vi "StateMachine.vi"() -> ()   [LabVIEW 2017]
uses:
  StateMachineControl.ctl
  global_output.vi
  IR_global.vi
  global_stop.vi
panel:
  in  "Go":bool
  out "State":T1
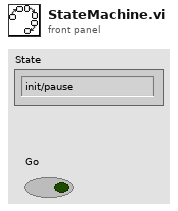
[diagram p1: front panel]
types:
  T1 = typedef "StateMachineControl.ctl" = enum16{"init/pause", "waypoint A", "wait at A", "waypoint B", "wait at B"}
  T2 = typedef "StateMachineControl.ctl" = enum16{"init/pause", "forward", "left", "right", "continue left", "continue right", "shutdown"}
  T3 = enum16{"Forward", "Backward", "Left", "Right", "Rotate Left", "Rotate Right"}
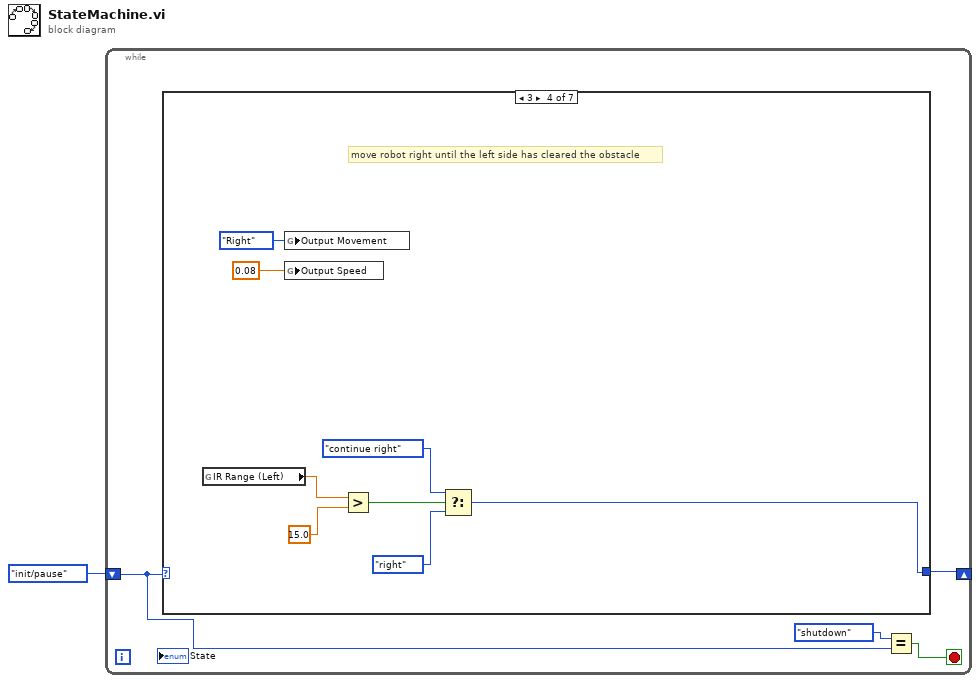
[diagram p0: block diagram]
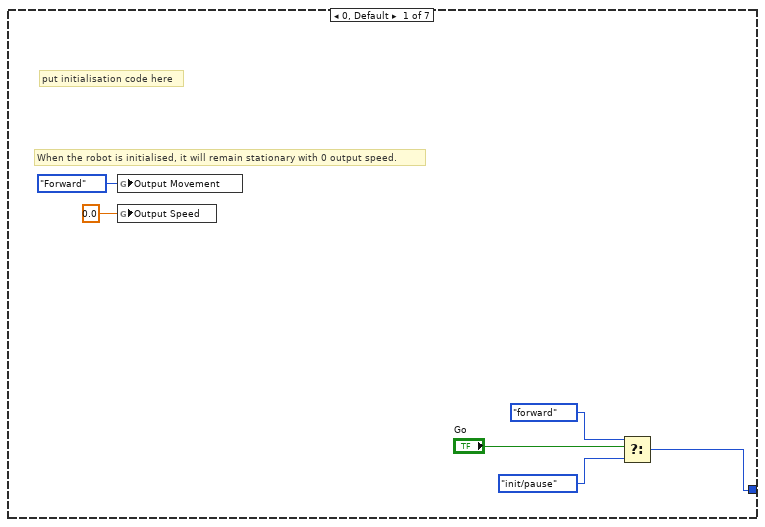
[diagram p2: hidden frame]
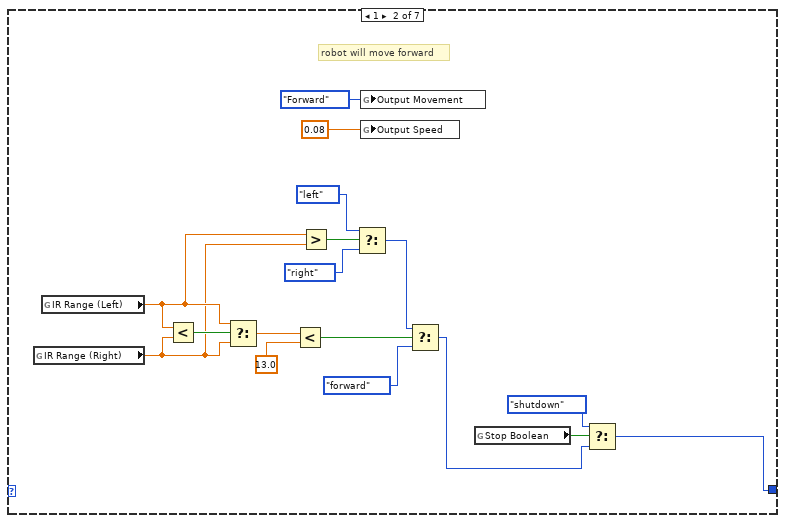
[diagram p3: hidden frame]
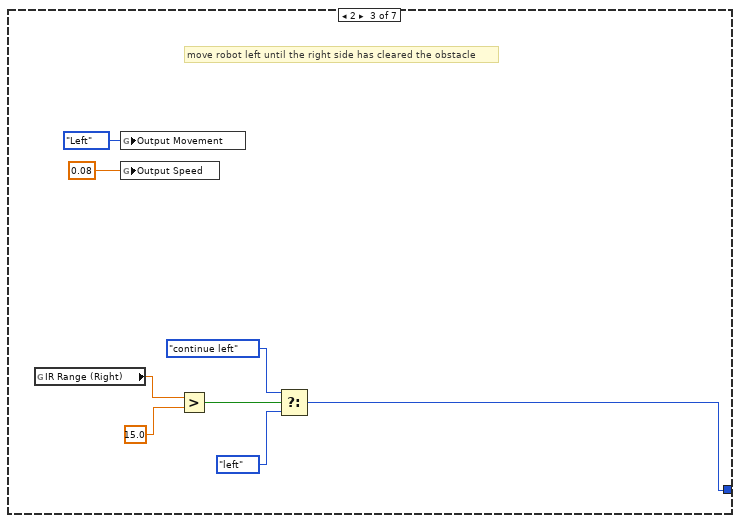
[diagram p4: hidden frame]
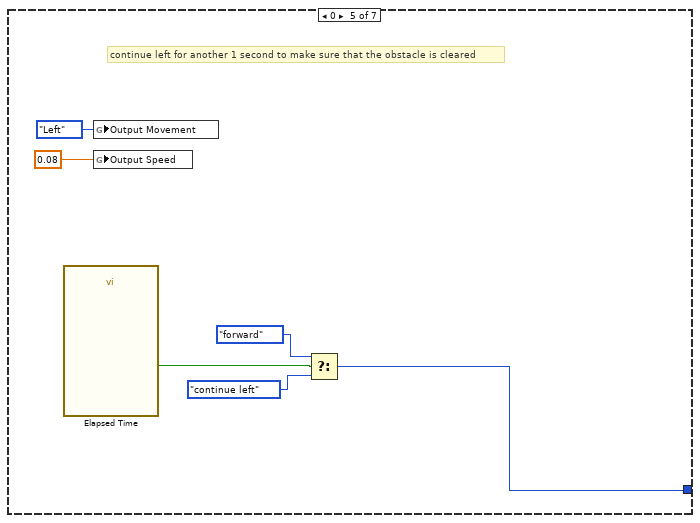
[diagram p5: hidden frame]
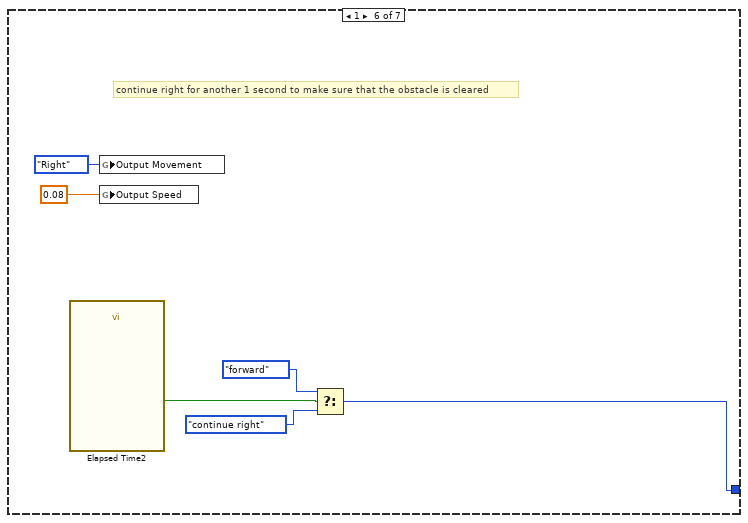
[diagram p6: hidden frame]
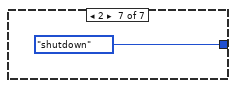
[diagram p7: hidden frame]
diagram:
  n1 = while {
    shift-right: [w5] -> _
    shift-left: StateMachineControl."init/pause" ("State") -> [w3]
    stop <- w2 stop-if-true
    n2 = case shown="3" w3 {
      tunnel: [w6 w14 w29 w37 w45 w51 StateMachineControl."shutdown" ("State")] -> w5
      frame 0, Default {
        # "When the robot is initialised, it will remain stationary with 0 output speed."
        # "put initialisation code here"
        n3 = global write "global_output.vi" "Output Movement"(T3."Forward" ("Output Movement")) -> ()
        n4 = global write "global_output.vi" "Output Speed"(0.0 ("Output Speed")) -> ()
        n5 = Select(t=StateMachineControl."forward" ("State"), s="Go", f=StateMachineControl."init/pause" ("State")) -> (s? t:f=w6:u16)
      }
      frame 1 {
        # "robot will move forward"
        n6 = global read "IR_global.vi" "IR Range (Right)"() -> (w23:dbl)
        n7 = global read "IR_global.vi" "IR Range (Left)"() -> (w24:dbl)
        n8 = Less?(x=w24, y=w23) -> (x < y?=w28:bool)
        n9 = Select(t=w24, s=w28, f=w23) -> (s? t:f=w27:dbl)
        n10 = Less?(x=w27, y=13.0) -> (x < y?=w25:bool)
        n11 = Greater?(x=w24, y=w23) -> (0:w22:bool)
        n12 = Select(t=StateMachineControl."left" ("State"), s=w22, f=StateMachineControl."right" ("State")) -> (s? t:f=w19:T2)
        n13 = global write "global_output.vi" "Output Movement"(T3."Forward" ("Output Movement")) -> ()
        n14 = global write "global_output.vi" "Output Speed"(0.08 ("Output Speed")) -> ()
        n15 = Select(t=w19, s=w25, f=StateMachineControl."forward" ("State")) -> (s? t:f=w15:T2)
        n16 = global read "global_stop.vi" "Stop Boolean"() -> (w17:bool)
        n17 = Select(t=StateMachineControl."shutdown" ("State"), s=w17, f=w15) -> (s? t:f=w14:T2)
      }
      frame 2 {
        # "move robot left until the right side has cleared the obstacle"
        n18 = global read "IR_global.vi" "IR Range (Right)"() -> (w34:dbl)
        n19 = global write "global_output.vi" "Output Movement"(T3."Left" ("Output Movement")) -> ()
        n20 = global write "global_output.vi" "Output Speed"(0.08 ("Output Speed")) -> ()
        n21 = Greater?(x=w34, y=15.0) -> (0:w32:bool)
        n22 = Select(t=StateMachineControl."continue left" ("State"), s=w32, f=StateMachineControl."left" ("State")) -> (s? t:f=w29:T2)
      }
      frame 3 {
        # "move robot right until the left side has cleared the obstacle"
        n23 = global read "IR_global.vi" "IR Range (Left)"() -> (w42:dbl)
        n24 = global write "global_output.vi" "Output Movement"(T3."Right" ("Output Movement")) -> ()
        n25 = global write "global_output.vi" "Output Speed"(0.08 ("Output Speed")) -> ()
        n26 = Greater?(x=w42, y=15.0) -> (0:w40:bool)
        n27 = Select(t=StateMachineControl."continue right" ("State"), s=w40, f=StateMachineControl."right" ("State")) -> (s? t:f=w37:T2)
      }
      frame 0 {
        # "continue left for another 1 second to make sure that the obstacle is cleared"
        n28 = call "Elapsed Time"() -> ("Time has Elapsed"=w48:bool)  [unwired: 12 in, 7 out]
        n29 = global write "global_output.vi" "Output Movement"(T3."Left" ("Output Movement")) -> ()
        n30 = global write "global_output.vi" "Output Speed"(0.08 ("Output Speed")) -> ()
        n31 = Select(t=StateMachineControl."forward" ("State"), s=w48, f=StateMachineControl."continue left" ("State")) -> (s? t:f=w45:T2)
      }
      frame 1 {
        # "continue right for another 1 second to make sure that the obstacle is cleared"
        n32 = call "Elapsed Time2"() -> ("Time has Elapsed"=w54:bool)  [unwired: 12 in, 7 out]
        n33 = global write "global_output.vi" "Output Movement"(T3."Right" ("Output Movement")) -> ()
        n34 = global write "global_output.vi" "Output Speed"(0.08 ("Output Speed")) -> ()
        n35 = Select(t=StateMachineControl."forward" ("State"), s=w54, f=StateMachineControl."continue right" ("State")) -> (s? t:f=w51:T2)
      }
      frame 2 {
      }
    }
    n36 = Equal?(x=StateMachineControl."shutdown" ("State"), y=w3) -> (x = y?=w2:bool)
  }
